vi "Auti LIN Do Polynom.vi"(6 "Polynomkoeff.":dbl[](array[numeric]), 8 "error in (no error)":errorcluster caption="Fehler (Eingang, kein Fehler)", 9 "Sollwerte":dbl[](array[numeric]), 10 "Rohwerte":dbl[](array[numeric]), 11 "Eingabetabelle":T1) -> (0 "error out":errorcluster caption="Fehler (Ausgang)", 2 "Tabelle":string[][](array[string]), 3 "Linearisiert":dbl[](array[numeric]))   [LabVIEW 2020, in "Linearisierung v2.lvlib"]
uses:
  Linearisierung v2.lvlib
  Eingabetabelle.ctl
  AutoLin Protokoll/AutoLin Protokoll.lvlib
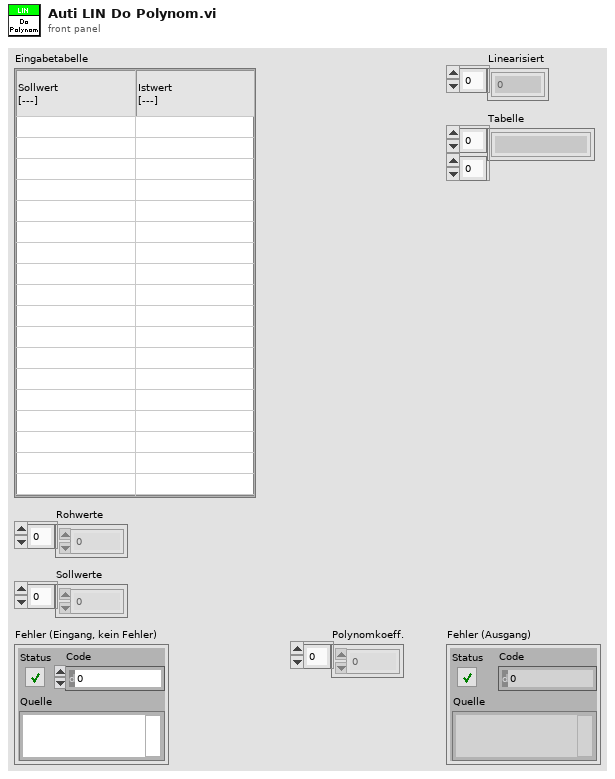
[diagram p1: front panel]
types:
  T1 = typedef "Linearisierung v2.lvlib/Eingabetabelle.ctl" = string[][]
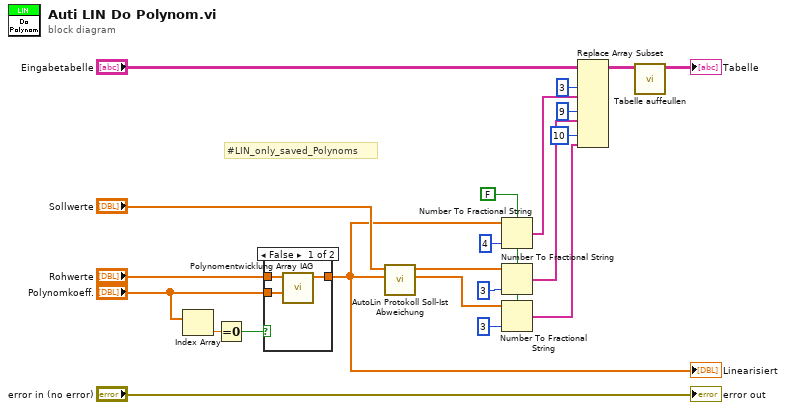
[diagram p0: block diagram]
diagram:
  w22 = FALSE ("Systemdezimalzeichen verwenden (T)")
  # "#LIN_only_saved_Polynoms"
  n1 = Index Array(array="Polynomkoeff.") -> (element=w4:dbl)  [unwired: 1 in]
  n2 = Equal To 0?(x=w4) -> (x = 0?=w3:bool)
  n3 = case shown="False" w3 {
    tunnel: "Polynomkoeff." -> [w25 _]
    tunnel: "Rohwerte" -> [w24 w26]
    tunnel: [w23 w26] -> w8
    frame False {
      n4 = call "Polynomentwicklung Array IAG.vi"("P(x) 2"=w25, "A"=w24) -> ("P(A)"=w23:dbl[])  [unwired: 9 in]
    }
    frame True {
    }
  }
  "Linearisiert" <- w8
  n5 = call "AutoLin Protokoll Soll-Ist Abweichung.vi"("Istwerte (ppm)"=w8, "Sollwerte (ppm)"="Sollwerte") -> ("% vom Sollwert"=w10:sgl[], "abs. Fehler (ppm)"=w9:sgl[])  [unwired: 7 in, 1 out]
  n6 = Number To Fractional String(use system decimal point (T)=w22, number=w8, precision (6)=i16 4 ("Genauigkeit (6)")) -> (F-format string=w11:string[])  [unwired: 1 in]
  n7 = Number To Fractional String(use system decimal point (T)=w22, number=w9, precision (6)=i16 3 ("Genauigkeit (6)")) -> (F-format string=w13:string[])  [unwired: 1 in]
  n8 = Number To Fractional String(use system decimal point (T)=w22, number=w10, precision (6)=i16 3 ("Genauigkeit (6)")) -> (F-format string=w15:string[])  [unwired: 1 in]
  n9 = Replace Array Subset(array="Eingabetabelle", new element #1=w11, index (col) #1=3 ("Deaktivierter Index (Spalte)"), new element #2=w13, index (col) #2=9 ("Index (Spalte)"), new element #3=w15, index (col) #3=10 ("Index (Spalte)")) -> (w17:T1)  [unwired: 3 in]
  n10 = call "Tabelle auffeullen.vi"("Neue Tabelle"=w17) -> ("Tabelle"=→"Tabelle":string[][])  [unwired: 10 in]
  "error out" <- "error in (no error)"
